vi "Json Parse.vi"(8 "error in (no error)":errorcluster, 11 "JSON in":string) -> (0 "error out":errorcluster, 3 "variant":variant)   [LabVIEW 2024, in "WebView.lvclass"]
uses:
  WebView.lvclass
  WebView.lvclass/WebView.ctl
  System.Web.Extensions
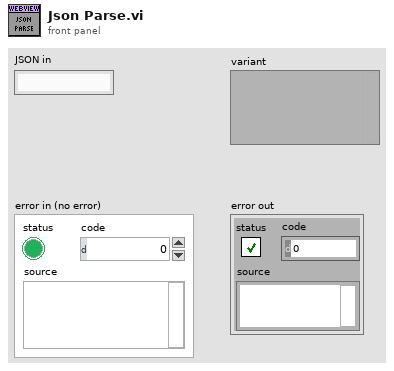
[diagram p1: front panel]
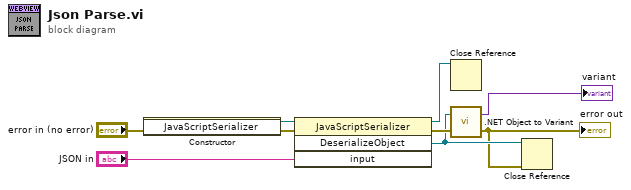
[diagram p0: block diagram]
diagram:
  n1 = constructor class="JavaScriptSerializer"(error in="error in (no error)") -> (reference out=w8:refnum<k24>, error out=w9:errorcluster)  [unwired: 2 in, 1 out]
  n2 = invoke class="JavaScriptSerializer" method="DeserializeObject"(reference=w8, error in=w9, "input"="JSON in") -> (reference out=w3:refnum<k24>, error out=w4:errorcluster, "DeserializeObject"=w2:refnum<k24>)  [unwired: 1 in, 1 out]
  n3 = Close Reference(reference=w3) -> ()  [unwired: 1 in, 1 out]
  n4 = call <vilib>:".NET Object to Variant.vi"("error in (no error)"=w4, ".NET object"=w2) -> ("error out"=w1:errorcluster, "variant"=→"variant":variant)
  "error out" <- w1
  n5 = Close Reference(reference=w2, error in (no error)=w1) -> ()  [unwired: 1 out]
